vi "CRYClose All Operator.vi"   [LabVIEW 2013]
uses:
  Misc/SubVI/CRYMisc vis settings global.vi
types:
  T1 = cluster{"Gen Idx":i32, "Chn Idx":i32, "Data":sgl[]}[]
  T2 = cluster{"Rcv Idx":i32, "Chn Idx":i32, "Data":i32[], "bufCount":i32}[]
  T3 = enum16{"OK", "Yes", "YesNo", "YesNoCancel", "ReplaceAppend"}
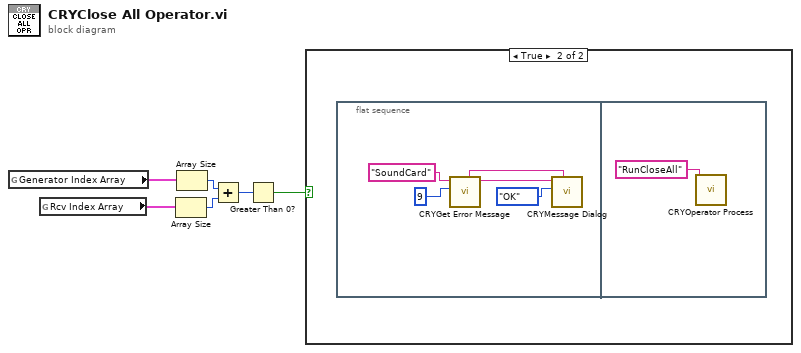
[diagram p0: block diagram]
diagram:
  n1 = global read "CRYMisc vis settings global.vi" "Generator Index Array"() -> (w6:T1)
  n2 = global read "CRYMisc vis settings global.vi" "Rcv Index Array"() -> (w5:T2)
  n3 = Array Size(array=w5) -> (size(s)=w3:i32)
  n4 = Array Size(array=w6) -> (size(s)=w4:i32)
  n5 = Add(x=w4, y=w3) -> (x+y=w2:i32)
  n6 = Greater Than 0?(x=w2) -> (x > 0?=w1:bool)
  n7 = case shown="True" w1 {
    frame False {
    }
    frame True {
      n8 = flat-sequence {
        frame #0 {
          n9 = call "CRYGet Error Message.vi"("Error No"=9, "Kind"="SoundCard") -> ("Message"=w10:string, "Window Title"=w9:string)  [unwired: 4 in, 4 out]
          n10 = call "CRYMessage Dialog.vi"("Window Title"=w9, "YesNoCancel"=T3."OK", "Message Content"=w10) -> ()  [unwired: 7 in, 2 out]
        }
        frame #1 {
          n11 = call "CRYOperator Process.vi"("sAction"="RunCloseAll") -> ()  [unwired: 10 in, 1 out]
        }
      }
    }
  }
